vi "button commands.vi"(6 "Buttons":T2, 7 "button info":T1, 9 "M3 Steps":dbl, 10 "M2 Steps":dbl, 11 "M1 Steps":dbl) -> (0 "Choose Button":bool, 1 "M3 distance":dbl, 2 "M2 distance":dbl, 3 "M1 distance":dbl)   [LabVIEW 2012]
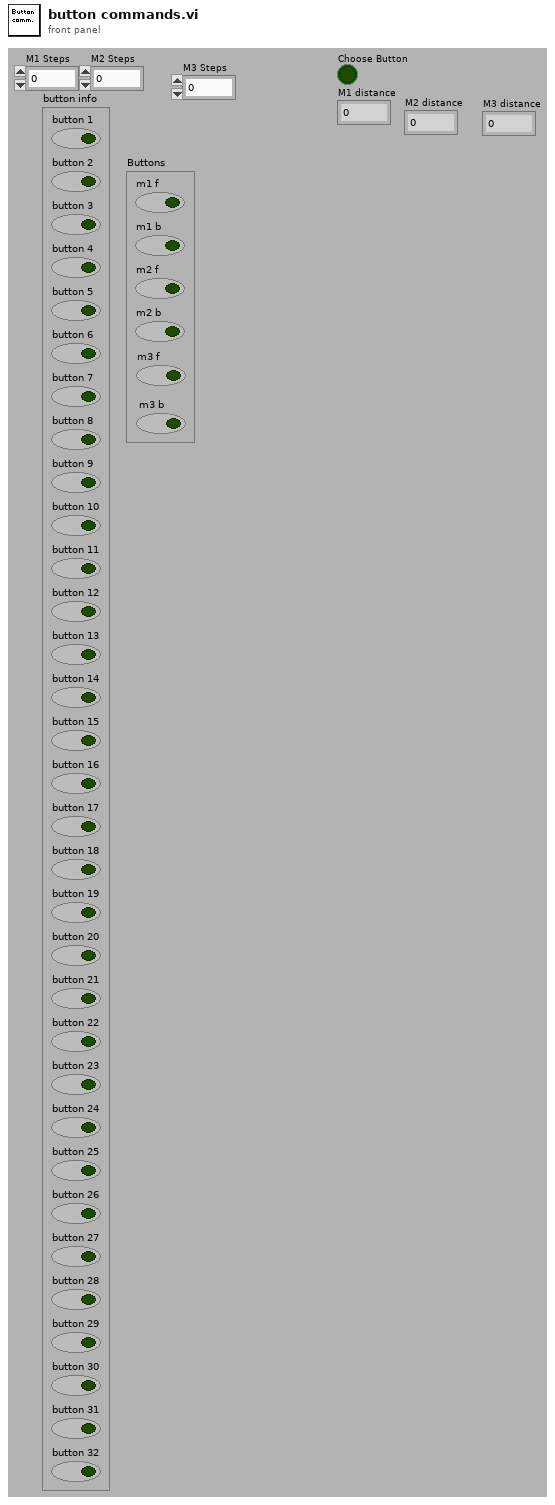
[diagram p1: front panel]
types:
  T1 = cluster{"button 1":bool, "button 2":bool, "button 3":bool, "button 4":bool, "button 5":bool, "button 6":bool, "button 7":bool, "button 8":bool, "button 9":bool, "button 10":bool, "button 11":bool, "button 12":bool, "button 13":bool, "button 14":bool, "button 15":bool, "button 16":bool, "button 17":bool, "button 18":bool, "button 19":bool, "button 20":bool, "button 21":bool, "button 22":bool, "button 23":bool, "button 24":bool, "button 25":bool, "button 26":bool, "button 27":bool, "button 28":bool, "button 29":bool, "button 30":bool, "button 31":bool, "button 32":bool}
  T2 = cluster{"m1 f":bool, "m1 b":bool, "m2 f":bool, "m2 b":bool, "m3 f":bool, "m3 b":bool}
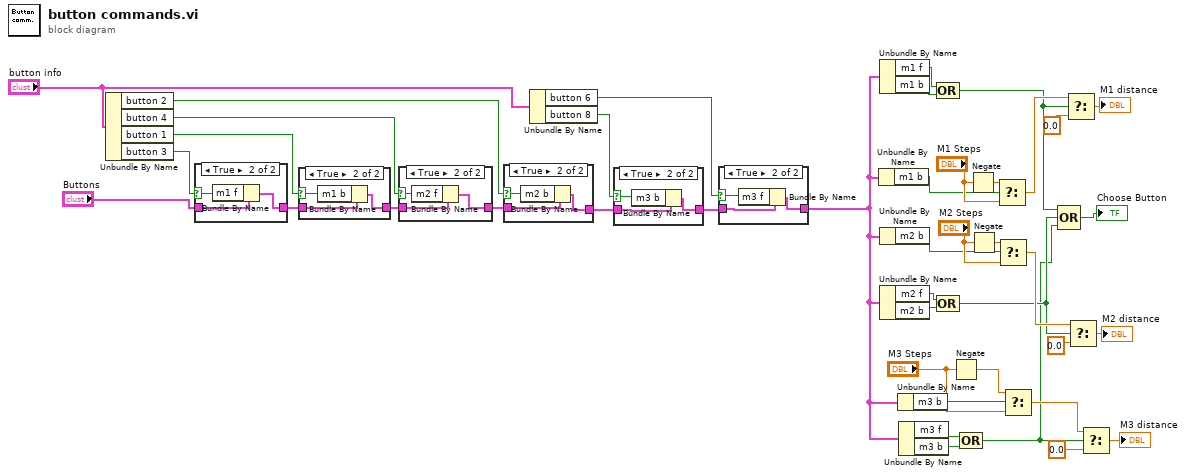
[diagram p0: block diagram]
diagram:
  n1 = Unbundle By Name("button info") -> ("button 2"=w20:bool, "button 4"=w21:bool, "button 1"=w22:bool, "button 3"=w23:bool)
  n2 = case shown="True" w23 {
    selector: w23 -> [_ w44]
    tunnel: "Buttons" -> [w43 w46]
    tunnel: [w43 w45] -> w24
    frame False {
    }
    frame True {
      n3 = Bundle By Name(cluster=w46, "m1 f"=w44) -> (w45:T2)
    }
  }
  n4 = case shown="True" w22 {
    selector: w22 -> [_ w48]
    tunnel: [w47 w50] -> w25
    tunnel: w24 -> [w47 w49]
    frame False {
    }
    frame True {
      n5 = Bundle By Name(cluster=w49, "m1 b"=w48) -> (w50:T2)
    }
  }
  n6 = case shown="True" w21 {
    selector: w21 -> [_ w52]
    tunnel: [w51 w54] -> w26
    tunnel: w25 -> [w51 w53]
    frame False {
    }
    frame True {
      n7 = Bundle By Name(cluster=w53, "m2 f"=w52) -> (w54:T2)
    }
  }
  n8 = case shown="True" w20 {
    selector: w20 -> [_ w56]
    tunnel: [w55 w58] -> w10
    tunnel: w26 -> [w55 w57]
    frame False {
    }
    frame True {
      n9 = Bundle By Name(cluster=w57, "m2 b"=w56) -> (w58:T2)
    }
  }
  n10 = Unbundle By Name("button info") -> ("button 6"=w6:bool, "button 8"=w7:bool)
  n11 = case shown="True" w7 {
    selector: w7 -> [_ w60]
    tunnel: w10 -> [w59 w61]
    tunnel: [w59 w62] -> w9
    frame False {
    }
    frame True {
      n12 = Bundle By Name(cluster=w61, "m3 b"=w60) -> (w62:T2)
    }
  }
  n13 = case shown="True" w6 {
    selector: w6 -> [_ w66]
    tunnel: w9 -> [w63 w65]
    tunnel: [w63 w64] -> w8
    frame False {
    }
    frame True {
      n14 = Bundle By Name(cluster=w65, "m3 f"=w66) -> (w64:T2)
    }
  }
  n15 = Unbundle By Name(w8) -> ("m1 b"=w4:bool)
  n16 = Unbundle By Name(w8) -> ("m1 f"=w36:bool, "m1 b"=w35:bool)
  n17 = Unbundle By Name(w8) -> ("m2 b"=w3:bool)
  n18 = Unbundle By Name(w8) -> ("m2 f"=w38:bool, "m2 b"=w37:bool)
  n19 = Unbundle By Name(w8) -> ("m3 b"=w15:bool)
  n20 = Unbundle By Name(w8) -> ("m3 f"=w17:bool, "m3 b"=w18:bool)
  n21 = Compound Arithmetic op=OR(w36, w35) -> (w28:bool)
  n22 = Compound Arithmetic op=OR(w38, w37) -> (w2:bool)
  n23 = Negate(x="M3 Steps") -> (-x=w12:dbl)
  n24 = Compound Arithmetic op=OR(w17, w18) -> (w1:bool)
  n25 = Negate(x="M1 Steps") -> (-x=w42:dbl)
  n26 = Negate(x="M2 Steps") -> (-x=w40:dbl)
  n27 = Select(t=w42, s=w4, f="M1 Steps") -> (s? t:f=w32:dbl)
  n28 = Select(t=w40, s=w3, f="M2 Steps") -> (s? t:f=w34:dbl)
  n29 = Select(t=w12, s=w15, f="M3 Steps") -> (s? t:f=w14:dbl)
  n30 = Compound Arithmetic op=OR(w28, w2, w1) -> (→"Choose Button":bool)
  n31 = Select(t=w32, s=w28, f=0.0) -> (s? t:f=→"M1 distance":dbl)
  n32 = Select(t=w34, s=w2, f=0.0) -> (s? t:f=→"M2 distance":dbl)
  n33 = Select(t=w14, s=w1, f=0.0) -> (s? t:f=→"M3 distance":dbl)
